vi "take_2_images_sbig.vi"(1 "Exptime":dbl, 2 "secondary path":path, 3 "primary_path":path) -> (0 "error out":errorcluster)   [LabVIEW 2018]
panel:
  out "appended path 2":path
  out "appended path":path
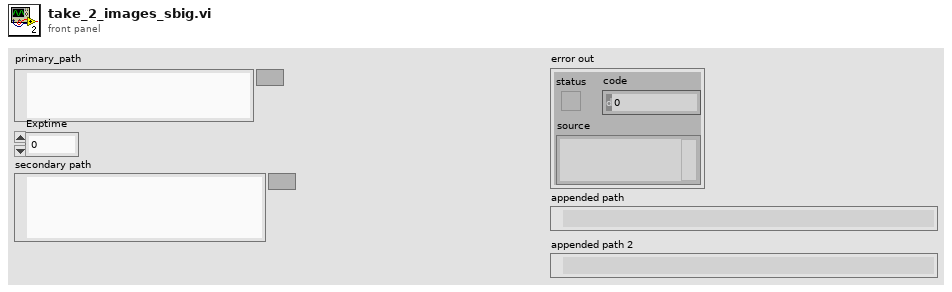
[diagram p1: front panel]
types:
  T1 = enum16{"open", "replace", "create", "open or create", "replace or create", "replace or create with confirmation"}
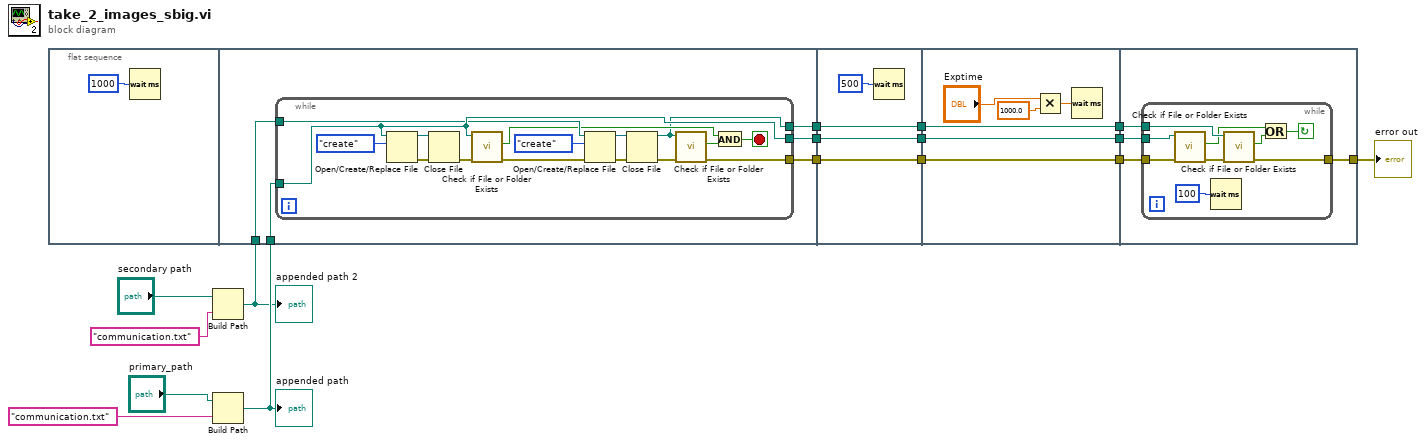
[diagram p0: block diagram]
diagram:
  n1 = flat-sequence {
    tunnel: w14 -> [w22]
    tunnel: [w21] -> w13
    tunnel: [w20] -> w12
    tunnel: w5 -> [w19]
    tunnel: [w18] -> w3
    tunnel: [w41] -> w10
    tunnel: w13 -> [w41]
    tunnel: [w40] -> w9
    tunnel: w12 -> [w40]
    tunnel: w3 -> [w39]
    tunnel: [w39] -> w2
    tunnel: [w45] -> w8
    tunnel: w10 -> [w45]
    tunnel: [w44] -> w7
    tunnel: w9 -> [w44]
    tunnel: w2 -> [w43]
    tunnel: [w43] -> w1
    tunnel: w8 -> [w52]
    tunnel: w7 -> [w51]
    tunnel: [w50] -> w11
    tunnel: w1 -> [w49]
    frame #0 {
      n2 = Wait (ms)(milliseconds to wait=u32 1000) -> ()  [unwired: 1 out]
    }
    frame #1 {
      n3 = while {
        tunnel: w22 -> [w37]
        tunnel: [w37] -> w21
        tunnel: [w32] -> w20
        tunnel: w19 -> [w34]
        tunnel: [w23] -> w18
        stop <- w29 stop-if-true
        n4 = Open/Create/Replace File(file path (use dialog)=w37, operation (0:open)=T1."create") -> (refnum out=w38:refnum<file>, error out=w28:errorcluster)  [unwired: 4 in, 1 out]
        n5 = Close File(refnum=w38, error in=w28) -> (error out=w27:errorcluster)  [unwired: 1 out]
        n6 = call <vilib>:"Check if File or Folder Exists.vi"("error in (no error)"=w27, "path"=w37) -> ("error out"=w26:errorcluster, "file or folder exists?"=w30:bool)  [unwired: 7 in, 1 out]
        n7 = Open/Create/Replace File(file path (use dialog)=w34, error in=w26, operation (0:open)=T1."create") -> (refnum out=w33:refnum<file>, error out=w25:errorcluster)  [unwired: 3 in, 1 out]
        n8 = Close File(refnum=w33, error in=w25) -> (path=w23:path, error out=w24:errorcluster)
        n9 = call <vilib>:"Check if File or Folder Exists.vi"("error in (no error)"=w24, "path"=w23) -> ("error out"=w32:errorcluster, "file or folder exists?"=w31:bool)  [unwired: 7 in, 1 out]
        n10 = And(x=w30, y=w31) -> (x .and. y?=w29:bool)
      }
    }
    frame #2 {
      n11 = Wait (ms)(milliseconds to wait=u32 500) -> ()  [unwired: 1 out]
    }
    frame #3 {
      n12 = Multiply(x="Exptime", y=1000.0) -> (x*y=w47:dbl)
      n13 = Wait (ms)(milliseconds to wait=w47) -> ()  [unwired: 1 out]
    }
    frame #4 {
      n14 = while {
        tunnel: w52 -> [w60]
        tunnel: w51 -> [w59]
        tunnel: [w56] -> w50
        tunnel: w49 -> [w58]
        stop <- w55 continue-if-true
        n15 = call <vilib>:"Check if File or Folder Exists.vi"("error in (no error)"=w59, "path"=w60) -> ("error out"=w57:errorcluster, "file or folder exists?"=w54:bool)  [unwired: 7 in, 1 out]
        n16 = Wait (ms)(milliseconds to wait=u32 100) -> ()  [unwired: 1 out]
        n17 = call <vilib>:"Check if File or Folder Exists.vi"("error in (no error)"=w57, "path"=w58) -> ("error out"=w56:errorcluster, "file or folder exists?"=w53:bool)  [unwired: 7 in, 1 out]
        n18 = Or(x=w54, y=w53) -> (x .or. y?=w55:bool)
      }
    }
  }
  n19 = Build Path(base path="secondary path", name or relative path="communication.txt") -> (appended path=w5:path)
  "appended path 2" <- w5
  n20 = Build Path(base path="primary_path", name or relative path="communication.txt") -> (appended path=w14:path)
  "appended path" <- w14
  "error out" <- w11
